vi "Roller Step Eject.vi"() -> (0 "Close Rollers?":bool, 2 "Right Out":dbl, 3 "Left Out":dbl)   [LabVIEW 2014]
uses:
  Robot Global Data.vi
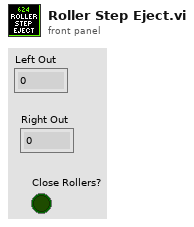
[diagram p1: front panel]
types:
  T1 = typedef "Dashboard Control Data.ctl" = cluster{"Cam Exposure":dbl, "Go to angle":dbl, "Steer PID Gains":cluster{"proportional gain (Kc)":dbl, "integral time (Ti, min)":dbl, "derivative time (Td, min)":dbl}, "Steer PID output Range":cluster{"output high":dbl, "output low":dbl}, "Pressure m \nValue":dbl, "Pressure b \nValue":dbl, "Roller Command Cluster ":T2, "Elevator":T3, "Encoder Control":T5, "IMU Controls":cluster{"Pitch Zero":dbl, "Roll Zero":dbl}, "Auton Settings":cluster{"Drive Dist Window Size":dbl}, "Drivetrain Settings":T6}
  T2 = typedef "Roller Control.ctl" = cluster{"Intake Speed":dbl, "Turn In Speed":dbl, "Unload Speed":dbl, "Turn Out Speed":dbl, "Ping Align Tolerance":dbl, "Tote Range Threshold":dbl, "Right Pot 0":dbl, "Pot Threshold":dbl, "Left Pot 0":dbl, "Manual 0s?":bool, "Right Pot Scale":dbl, "Left Pot Scale":dbl, "0 wait time":i32, "Zero Pots":bool, "Min Elevator Height":dbl, "Eject Time":dbl, "Eject US Threshold":dbl, "Anti-Twitch Time":u32, "Ping Caring Threshold":dbl, "Pot Diff Threshold":dbl, "Pinch Sustain":u32, "Absorb Give Up Threshold":dbl, "Untip In Threshold":dbl, "Untip Grab Range":dbl}
  T3 = typedef "Elevator DB Control.ctl" = cluster{"PID Output Range":cluster{"output high":dbl, "output low":dbl}, "PID gains":cluster{"proportional gain (Kc)":dbl, "integral time (Ti, min)":dbl, "derivative time (Td, min)":dbl}, "Height Tolerance":sgl, " Encoder Constant":dbl, "Safe Mode Max Speed":sgl, "Eject Time":sgl, "Zeroing Speed":sgl, "Presets":T4, "Ping Detect Threshold":sgl, "Trashcan Detect Threshold":sgl, "Zero Filter Time":dbl, "Stabilizer Open Time":dbl}
  T4 = typedef "Elevator Presets.ctl" = cluster{"Hold Tote":sgl, "Hold Trashcan":sgl, "Pickup 2 w/ Tote":sgl, "Pickup 2 w/ Trashcan":sgl, "Pickup 3 w/ Tote":sgl, "Pickup 3 w/ Trashcan":sgl, "Bottom":sgl, "Pickup 1 w/ Tote":sgl, "Pickup Trashcan":sgl, "Pickup 1 w/ Trashcan":sgl, "Eject":sgl, "Hold Low":sgl, "Step add height":sgl, "Store Trashcan 3":sgl, "Store Trashcan 4":sgl, "Store Trashcan 5":sgl, "6 Tote Max Height":sgl, "5 Tote Max Height":sgl, "Idle Empty":dbl, "Untip Lift":dbl, "Drop Stack":dbl}
  T5 = typedef "Encoder Control.ctl" = cluster{"Left Tick Constant":dbl, "Right Tick Constant":dbl, "Center Tick Constant":dbl, "Reset?":bool, "Y Dist":cluster{"PID gains":cluster{"proportional gain (Kc)":dbl, "integral time (Ti, min)":dbl, "derivative time (Td, min)":dbl}, "output range":cluster{"output high":dbl, "output low":dbl}}, "X Dist":cluster{"PID gains":cluster{"proportional gain (Kc)":dbl, "integral time (Ti, min)":dbl, "derivative time (Td, min)":dbl}, "output range":cluster{"output high":dbl, "output low":dbl}}, "Y Stop Thresh":dbl, "Y Stop Speed":dbl, "X Stop Thresh":dbl, "X Stop Speed":dbl}
  T6 = typedef "Drivetrain Settings.ctl" = cluster{"Gyro Tolerance":dbl, "Strafe Correct max steer":dbl, "Strafe Timer Wait":dbl}
  T7 = typedef "Elevator Status.ctl" = cluster{"Eject Piston":bool, "Height":dbl, "Top Limit":bool, "Bottom Limit":bool, "Enc Value":dbl, "Limit Override":bool, "Mode":T8, "Stabilizer":bool, "Finger":bool, "High IR":bool, "Motor Out":dbl, "Ping Detect":bool, "Auto Elevator Indicators":T9}
  T8 = typedef "Elevator Mode.ctl" = enum16{"Manual", "Safe", "Auto"}
  T9 = typedef "Auto Elevator Indicators.ctl" = cluster{"Target Out":dbl, "Storing Trashcan?":bool, "State":T10, "In Range":bool, "Store Can Command":bool}
  T10 = typedef "Elevator State.ctl" = enum16{"Idle", "Goto Load Position", "Wait for Load", "Load Drop", "Load Lift", "Drop Stack", "Goto Eject Position", "Eject ", "Raise Trashcan", "Open Stabilizer", "Untip Drop", "Untip Wait", "Untip Lift"}
  T11 = typedef "Ultrasonic Indicators.ctl" = cluster{"Left Distance":dbl, "Right Distance":dbl, "Center Distance":dbl}
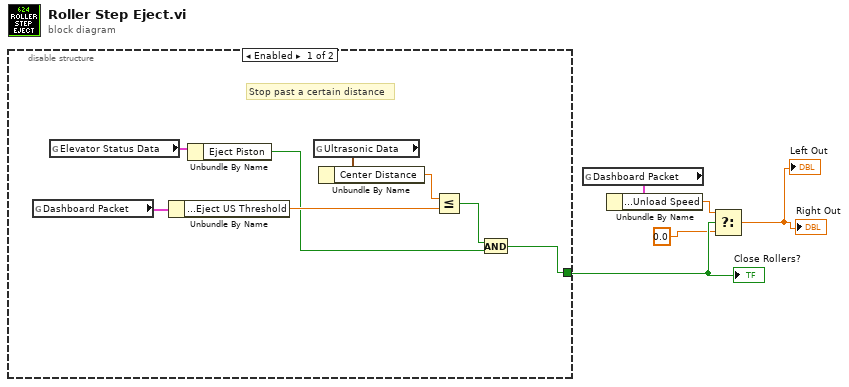
[diagram p0: block diagram]
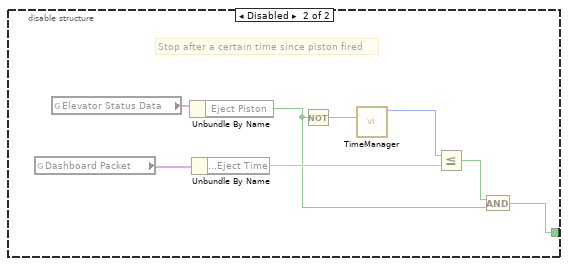
[diagram p2: hidden frame]
diagram:
  n1 = disable-structure shown="Enabled" {
    disable-tunnel: [w6 w14] -> w4
    frame Enabled {
      # "Stop past a certain distance"
      n2 = global read "Robot Global Data.vi" "Dashboard Packet"() -> (w12:T1)
      n3 = global read "Robot Global Data.vi" "Elevator Status Data"() -> (w13:T7)
      n4 = Unbundle By Name(w12) -> ("Roller Command Cluster.Eject US Threshold"=w11:dbl)
      n5 = Unbundle By Name(w13) -> ("Eject Piston"=w9:bool)
      n6 = global read "Robot Global Data.vi" "Ultrasonic Data"() -> (w8:T11)
      n7 = Unbundle By Name(w8) -> ("Center Distance"=w7:dbl)
      n8 = Less Or Equal?(x=w7, y=w11) -> (x <= y?=w10:bool)
      n9 = And(x=w10, y=w9) -> (x .and. y?=w6:bool)
    }
    frame Disabled {
      # "Stop after a certain time since piston fired"
      n10 = global read "Robot Global Data.vi" "Dashboard Packet"() -> (w18:T1)
      n11 = global read "Robot Global Data.vi" "Elevator Status Data"() -> (w20:T7)
      n12 = Unbundle By Name(w20) -> ("Eject Piston"=w15:bool)
      n13 = Unbundle By Name(w18) -> ("Roller Command Cluster.Eject Time"=w17:dbl)
      n14 = Not(x=w15) -> (.not. x?=w21:bool)
      n15 = call "TimeManager.vi"("Reset?"=w21) -> ("Time Since Reset"=w19:u32)  [unwired: 9 in, 1 out]
      n16 = Less Or Equal?(x=w19, y=w17) -> (x <= y?=w16:bool)
      n17 = And(x=w16, y=w15) -> (x .and. y?=w14:bool)
    }
  }
  "Close Rollers?" <- w4
  n18 = global read "Robot Global Data.vi" "Dashboard Packet"() -> (w5:T1)
  n19 = Unbundle By Name(w5) -> ("Roller Command Cluster.Unload Speed"=w3:dbl)
  n20 = Select(t=w3, s=w4, f=0.0) -> (s? t:f=→"Left Out" →"Right Out":dbl)
